vi "Read Child XML Node.vi"(8 "error in (no error)":errorcluster, 11 "Array in":refnum<class "Array.lvclass">) -> (0 "error out":errorcluster, 2 "Child XML Node":refnum<k20>, 3 "Array out":refnum<class "Array.lvclass">)   [LabVIEW 2025, in "Array.lvclass"]
uses:
  Array.lvclass
  Array.lvclass/Array.ctl
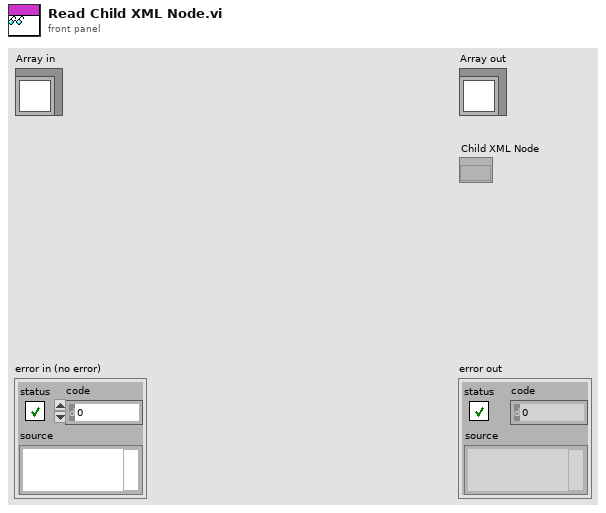
[diagram p1: front panel]
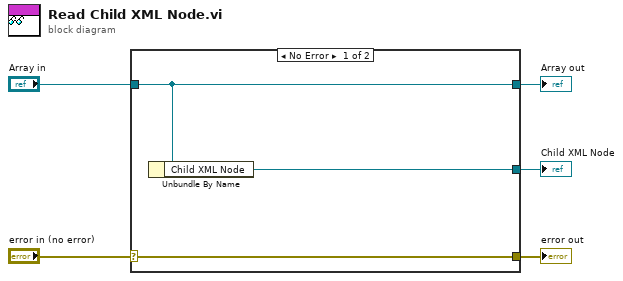
[diagram p0: block diagram]
diagram:
  n1 = case shown="No Error" "error in (no error)" {
    selector: "error in (no error)" -> [w8 w9]
    tunnel: [w8 w9] -> w4
    tunnel: [w7 w10] -> w2
    tunnel: "Array in" -> [w7 w10]
    tunnel: [w6 _] -> w1
    frame No Error {
      n2 = Unbundle By Name(w7) -> ("Child XML Node"=w6:refnum<k20>)
    }
    frame Error {
    }
  }
  "error out" <- w4
  "Array out" <- w2
  "Child XML Node" <- w1
